vi "PH_Beckhoff_PP_Control.ProcPeriodic.vi"(0 "i ref in":refnum<vi>, 3 "ms timeout (10000)":i32=10000, 5 "error in (no error)":errorcluster) -> (14 "i ref out":refnum<vi>, 17 "timed out":bool, 19 "error out":errorcluster)   [LabVIEW 2014, in "PH_Beckhoff_PP_Control.lvlib"]
doc: "This method serves to periodically do things like reading values from the HW. Methods that should be executed periodically should be called from THIS methode. Add code here."
uses:
  PH_Beckhoff_PP_Control.lvlib
  PH_Beckhoff/PH_Beckhoff.lvlib
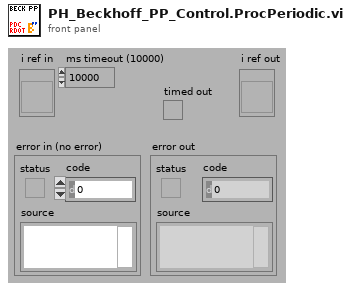
[diagram p1: front panel]
types:
  T1 = typedef "PH_Beckhoff.lvlib/PH_Beckhoff.i attribute.ctl" = cluster{"GUI Refs":T2, "operation?":bool, "Default Prdc Interval":i32, "Connection":T3, "AMS Net ID":T4, "Klemmencluster: # of":T5, "Values":T6, "IP":string, "Description":string, "configured?":bool, "Change Manager":cluster{"Detemination wanted?":bool, "Values changed at":cluster{"Sonderklemmen Inputs":i32[], "Analog Inputs":i32[], "Analog Outputs":i32[], "Digital Inputs":i32[], "Digital Outputs":i32[]}}, "Difference to handle an analog input as change":u32}
  T2 = typedef "PH_Beckhoff.lvlib/PH_Beckhoff.GUI Refs.ctl" = cluster{"ADS Error":refnum<vi>, "Values":refnum<vi>, "configured?":refnum<vi>, "Connection":refnum<vi>, "IP":refnum<vi>, "Prdc Int [ms]":refnum<vi>}
  T3 = typedef "PH_Beckhoff.lvlib/PH_Beckhoff.Connectivity.ctl" = cluster{"DLL?":bool, "Port?":bool, "Client?":bool, "Ping?":bool, "unsuccessful Pings":u32}
  T4 = typedef "Beckhoff - Driver np.lvlib/Beckhoff Access.ctl" = cluster{"DLL path":path, "AMS Net ID":cluster{"1st # of IP":u8, "2nd # of IP":u8, "3rd # of IP":u8, "4th # of IP":u8, "In Port":u8, "Out Port":u8}}
  T5 = typedef "Beckhoff - Driver np.lvlib/Klemmendeclarer.ctl" = cluster{"Offset due to Sonderklemms":u32, "analog Inputs":u32, "analog Outputs":u32, "digital Input Bits":u32, "digital Output Bits":u32}
  T6 = typedef "PH_Beckhoff.lvlib/PH_Beckhoff.Values.ctl" = cluster{"Sonderklemmen Inputs":T7, "Analog Inputs":T8, "Analog Outputs":T10, "Digital Inputs":T11, "Digital Outputs":T12}
  T7 = typedef "PH_Beckhoff.lvlib/PH_Beckhoff.Sonderklemmen Inputs.ctl" = cluster{"Total Length":u32, "Name":string, "Value":u64, "Quality":bool, "Service ID":i32, "Offset":u32, "Length":u32}[]
  T8 = typedef "PH_Beckhoff.lvlib/PH_Beckhoff.Analog Inputs.ctl" = cluster{"Name":string, "Value":u32, "Quality":bool, "Service ID":i32, "Sca Type":T9}[]
  T9 = typedef "PH_Beckhoff.lvlib/PH_Beckhoff.Scaling Type.ctl" = enum16{"none", "0 ... 15 Bit -> 0 ... 5", "0 ... 15 Bit -> 0 ... 10", "0 ... 15 Bit -> 0 ... 25", "0 ... 15 Bit -> 4 ... 20", "0 ... 15 Bit -> 0 ... 1", "0 ... 15 Bit -> 0 ... 20000", "0 ... 15 Bit -> 0 ... 24000"}
  T10 = typedef "PH_Beckhoff.lvlib/PH_Beckhoff.Analog Outputs.ctl" = cluster{"Name":string, "Value":u32, "Quality":bool, "Wanted Value":u32, "Service ID":i32, "Sca Type":T9}[]
  T11 = typedef "PH_Beckhoff.lvlib/PH_Beckhoff.Digital Inputs.ctl" = cluster{"Name":string, "Value":bool, "Quality":bool, "Service ID":i32, "inverted?":bool}[]
  T12 = typedef "PH_Beckhoff.lvlib/PH_Beckhoff.Digital Outputs.ctl" = cluster{"Name":string, "Value":bool, "Quality":bool, "Wanted Value":bool, "Service ID":i32, "inverted?":bool}[]
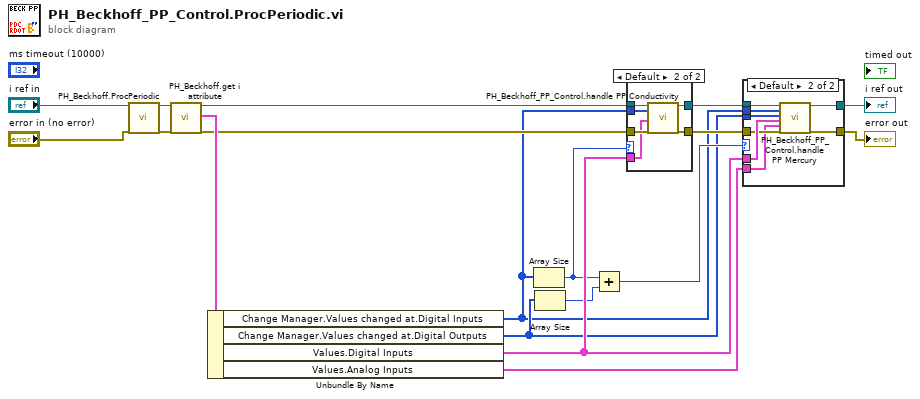
[diagram p0: block diagram]
diagram:
  n1 = call "PH_Beckhoff.ProcPeriodic.vi"("i ref in"="i ref in", "error in (no error)"="error in (no error)") -> ("i ref out"=w16:refnum<vi>, "error out"=w15:errorcluster)  [unwired: 15 in, 1 out]
  n2 = call "PH_Beckhoff.get i attribute.vi"("i ref in"=w16, "error in (no error)"=w15) -> ("i ref out"=w4:refnum<vi>, "i attribute"=w14:T1, "error out"=w3:errorcluster)  [unwired: 15 in]
  n3 = Unbundle By Name(w14) -> ("Change Manager.Values changed at.Digital Inputs"=w1:i32[], "Change Manager.Values changed at.Digital Outputs"=w2:i32[], "Values.Digital Inputs"=w10:T11, "Values.Analog Inputs"=w8:T8)
  n4 = Array Size(array=w1) -> (size(s)=w5:i32)
  n5 = Array Size(array=w2) -> (size(s)=w6:i32)
  n6 = Add(x=w5, y=w6) -> (x+y=w7:i32)
  n7 = case shown="Default" w5 {
    tunnel: w3 -> [w19 w26]
    tunnel: w4 -> [w20 w25]
    tunnel: [w20 w24] -> w13
    tunnel: w10 -> [_ w23]
    tunnel: [w19 w22] -> w9
    tunnel: w1 -> [_ w21]
    frame 0 {
    }
    frame Default {
      n8 = call "PH_Beckhoff_PP_Control.handle PP Conductivity.vi"("i ref in"=w25, "changed DE Values"=w21, "Current Digital Inputs"=w23, "error in"=w26) -> ("i ref out"=w24:refnum<vi>, "error out"=w22:errorcluster)  [unwired: 14 in]
    }
  }
  n9 = case shown="Default" w7 {
    tunnel: w13 -> [w28 w36]
    tunnel: [w28 w35] -> w12
    tunnel: [w27 w34] -> w11
    tunnel: w10 -> [_ w33]
    tunnel: w9 -> [w27 w32]
    tunnel: w8 -> [_ w31]
    tunnel: w2 -> [_ w30]
    tunnel: w1 -> [_ w29]
    frame 0 {
    }
    frame Default {
      n10 = call "PH_Beckhoff_PP_Control.handle PP Mercury.vi"("i ref in"=w36, "changed DE Values"=w29, "changed AE Values"=w30, "Current Digital Inputs"=w33, "Current Analog Inputs"=w31, "error in"=w32) -> ("i ref out"=w35:refnum<vi>, "error out"=w34:errorcluster)  [unwired: 12 in]
    }
  }
  "error out" <- w11
  "i ref out" <- w12
